vi "setLogString.vi"(8 "error in (no error)":errorcluster, 10 "logString":string, 11 "Log.lvclass in":refnum<class "Log.lvclass">) -> (0 "error out":errorcluster, 3 "Log.lvclass out":refnum<class "Log.lvclass">)   [LabVIEW 2011, in "Tools.lvlib" / "xml.lvlib" / "Log.lvclass"]
uses:
  Log.lvclass
  Log.lvclass/Log.ctl
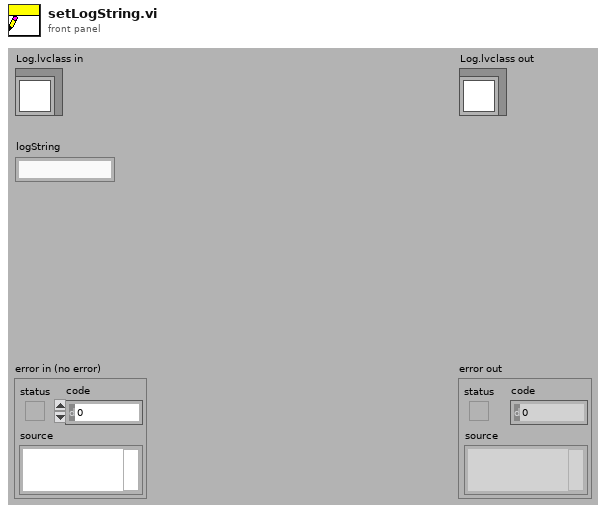
[diagram p1: front panel]
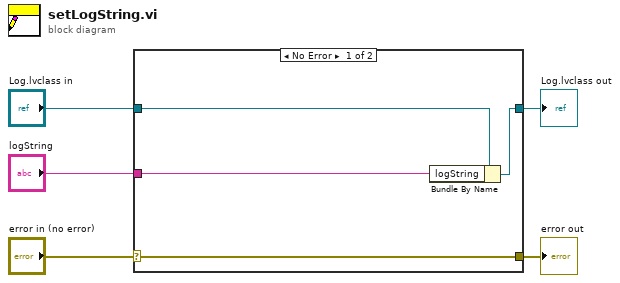
[diagram p0: block diagram]
diagram:
  n1 = case shown="No Error" "error in (no error)" {
    selector: "error in (no error)" -> [w9 w10]
    tunnel: [w9 w10] -> w4
    tunnel: [w7 w11] -> w2
    tunnel: "Log.lvclass in" -> [w8 w11]
    tunnel: "logString" -> [w6 _]
    frame No Error {
      n2 = Bundle By Name(cluster=w8, "logString"=w6) -> (w7:refnum<class "Log.lvclass">)
    }
    frame Error {
    }
  }
  "error out" <- w4
  "Log.lvclass out" <- w2
